vi "Create Control Queue Sensor910.vi"(8 "error in (no error)":errorcluster) -> (0 "error out":errorcluster, 1 "created new?":bool, 3 "queue out":refnum<queue>)   [LabVIEW 2020, in "Sensor910.lvclass"]
uses:
  Sensor910.lvclass
  Mode.ctl
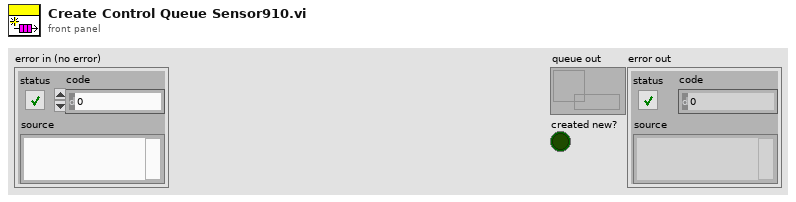
[diagram p1: front panel]
types:
  T1 = typedef "Sensor910.lvclass/Mode.ctl" = enum16{"Inactiv", "Read Data", "Service Mode", "Enter offset", "Open session", "Close session", "Set Modbus Address", "Abort"}
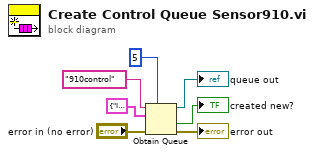
[diagram p0: block diagram]
diagram:
  n1 = Obtain Queue(max queue size (-1, unlimited)=5, name (unnamed)="910control", element data type=cluster{"Mode":T1, "Data":variant} {"Mode"=enum."Inactiv", "Data"=variant}, error in (no error)="error in (no error)") -> (queue out=→"queue out":refnum<queue>, created new?=→"created new?":bool, error out=→"error out":errorcluster)  [unwired: 1 in]
